vi "DC Responsivity.vi"() -> ()   [LabVIEW 2018]
uses:
  <vilib>/Analysis/baseanly.llb/Mean (DBL).vi
  <vilib>/express/express shared/transition.llb/Dynamic To Waveform Array.vi
  <vilib>/express/express signal manip/GetorSetDDTAttributes/Set DDT Attributes/SetT0.vi
  <vilib>/express/express shared/transition.llb/Waveform Array To Dynamic.vi
  <vilib>/express/express signal manip/GetorSetDDTAttributes/Set DDT Attributes/Set DDT Properties.xnode
  <vilib>/Analysis/NI_AALBase.lvlib
panel:
  in  "Enable":bool=TRUE
  in  "Filename":path=path "C:/Users/physics-svc-fulda/Desktop/LabVIEW Data/DC A.lvm"
  out "DC Offset A":dbl format="%0.6f"
  out "DC Offset C":dbl format="%0.6f"
  out "DC Offset B":dbl format="%0.6f"
  out "DC Offset D":dbl format="%0.6f"
  out "Quadrant Power":dynamicdata(graph)
  out "Saving Data":bool
  in  "Which Quadrant":string
  out "Max Power":dbl
  out "DC D":dbl format="%0.6f"
  out "DC C":dbl format="%0.6f"
  out "DC B":dbl format="%0.6f"
  out "DC A":dbl format="%0.6f"
  in  "timeout (s)":dbl=10.0 format="%0.2f"
  in  "rate":dbl=1000.0
  in  "# of samples":i32=100
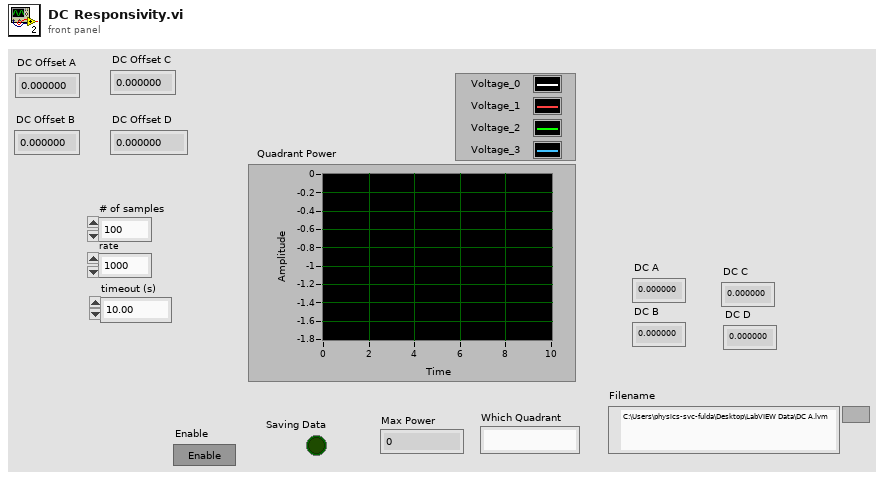
[diagram p1: front panel]
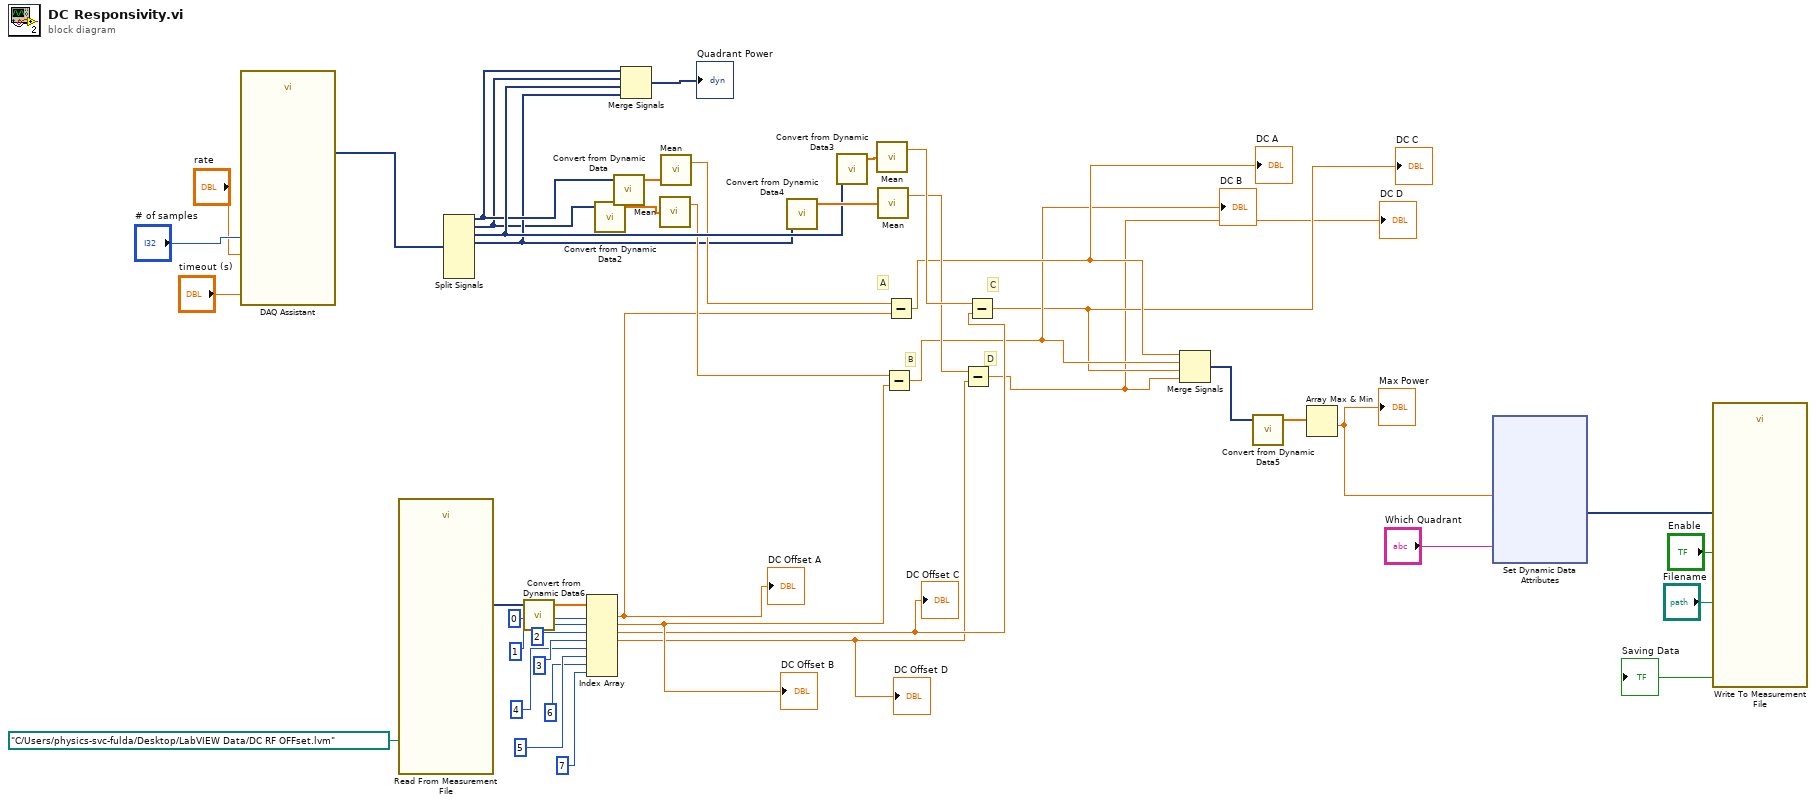
[diagram p0: block diagram]
diagram:
  # "D"
  # "B"
  # "C"
  # "A"
  n1 = call "DAQ Assistant"("rate"="rate", "number of samples"="# of samples", "timeout (s)"="timeout (s)") -> ("data"=w41:dynamicdata)  [unwired: 14 in, 2 out]
  n2 = call "Read From Measurement File"("Filename"=path "C:/Users/physics-svc-fulda/Desktop/LabVIEW Data/DC RF OFFset.lvm") -> ("Signals"=w22:dynamicdata)  [unwired: 5 in, 5 out]
  n3 = Split Signals(w41) -> (w24:dynamicdata, w8:dynamicdata, w31:dynamicdata, w23:dynamicdata)  [unwired: 8 in, 4 out]
  n4 = call "Convert from Dynamic Data6"("Dynamic Data Type"=w22) -> ("Array"=w21:dbl[])  [unwired: 3 in]
  n5 = Index Array(array=w21, index #1=0 ("index"), index #2=1 ("index"), index #3=2 ("index"), index #4=3 ("index"), index #5=4 ("index"), index #6=5 ("index"), index #7=6 ("index"), index #8=7 ("index")) -> (element #1=w12:dbl, element #2=w11:dbl, element #3=w10:dbl, element #4=w9:dbl)  [unwired: 4 out]
  "DC Offset D" <- w9
  "DC Offset B" <- w11
  "DC Offset C" <- w10
  "DC Offset A" <- w12
  n6 = call "Convert from Dynamic Data2"("Dynamic Data Type"=w8) -> ("Array"=w39:dbl[])  [unwired: 3 in]
  n7 = call "Convert from Dynamic Data"("Dynamic Data Type"=w24) -> ("Array"=w40:dbl[])  [unwired: 3 in]
  n8 = Merge Signals(w24, w8, w31, w23) -> (→"Quadrant Power":dynamicdata)
  n9 = call-poly <vilib>:"Mean.vi"("X"=w39) -> ("mean"=w27:dbl)  [unwired: 1 out]
  n10 = call-poly <vilib>:"Mean.vi"("X"=w40) -> ("mean"=w28:dbl)  [unwired: 1 out]
  n11 = call "Convert from Dynamic Data4"("Dynamic Data Type"=w23) -> ("Array"=w37:dbl[])  [unwired: 3 in]
  n12 = call "Convert from Dynamic Data3"("Dynamic Data Type"=w31) -> ("Array"=w38:dbl[])  [unwired: 3 in]
  n13 = call-poly <vilib>:"Mean.vi"("X"=w38) -> ("mean"=w26:dbl)  [unwired: 1 out]
  n14 = call-poly <vilib>:"Mean.vi"("X"=w37) -> ("mean"=w25:dbl)  [unwired: 1 out]
  n15 = Subtract(x=w27, y=w11) -> (x-y=w3:dbl)
  "DC B" <- w3
  n16 = Subtract(x=w28, y=w12) -> (x-y=w4:dbl)
  "DC A" <- w4
  n17 = Subtract(x=w25, y=w9) -> (x-y=w1:dbl)
  "DC D" <- w1
  n18 = Subtract(x=w26, y=w10) -> (x-y=w2:dbl)
  "DC C" <- w2
  n19 = Merge Signals(w4, w3, w2, w1) -> (w36:dynamicdata)
  n20 = call "Convert from Dynamic Data5"("Dynamic Data Type"=w36) -> ("Array"=w35:dbl[])  [unwired: 3 in]
  n21 = Array Max & Min(array=w35) -> (min value=w7:dbl)  [unwired: 3 out]
  "Max Power" <- w7
  n22 = xnode "Set Dynamic Data Attributes"("Signals In"=w7, "Signal Name"="Which Quadrant") -> ("Signals Out"=w32:dynamicdata)  [unwired: 2 in, 1 out]
  n23 = call "Write To Measurement File"("Signals"=w32, "Enable"="Enable", "Filename"="Filename") -> ("Saving Data"=→"Saving Data":bool)  [unwired: 14 in, 2 out]
